vi "Sample - Add Speciment (SubVI).vi"(6 "Load?":bool, 7 "ID":string, 8 "error in":errorcluster, 9 "Data":string[](array[string]), 11 "JobID":string) -> (0 "error in 2":errorcluster, 3 "body":string)   [LabVIEW 2019]
uses:
  <vilib>/httpClient/POSTBuffer.vi
  <vilib>/httpClient/LabVIEWHTTPClient.lvlib
panel:
  in  "Type":enum16{"Circular", "Cubical"}(ring) caption="Enum 3"
  in  "Save":bool
  in  "Weight (g)":dbl format="%.2f"
  in  "Diameter/Length (mm)":dbl format="%.2f"
  in  "Height (mm)":dbl format="%.2f"
  in  "Depth (m)":dbl format="%.2f"
  in  "Specimen No":string
  in  "Sample No":string
  # "Specimen Details"
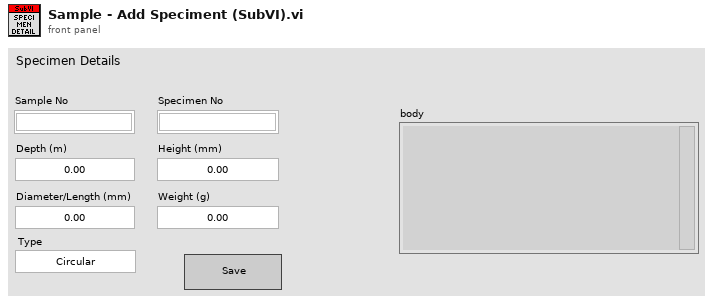
[diagram p1: front panel]
types:
  T1 = cluster{"action":string, "sampleno":string, "specimentno":string, "weight":string, "height":string, "depth":string, "diameter":string, "id":string, "jobid":string, "attribute":string}
  T2 = cluster{"action":string, "jobid":string, "sampleno":string, "specimentno":string, "weight":string, "height":string, "depth":string, "diameter":string, "attribute":string}
  T3 = typedef "LabVIEWHTTPClient.lvlib/ClientHandle.ctl" = refnum<k1>
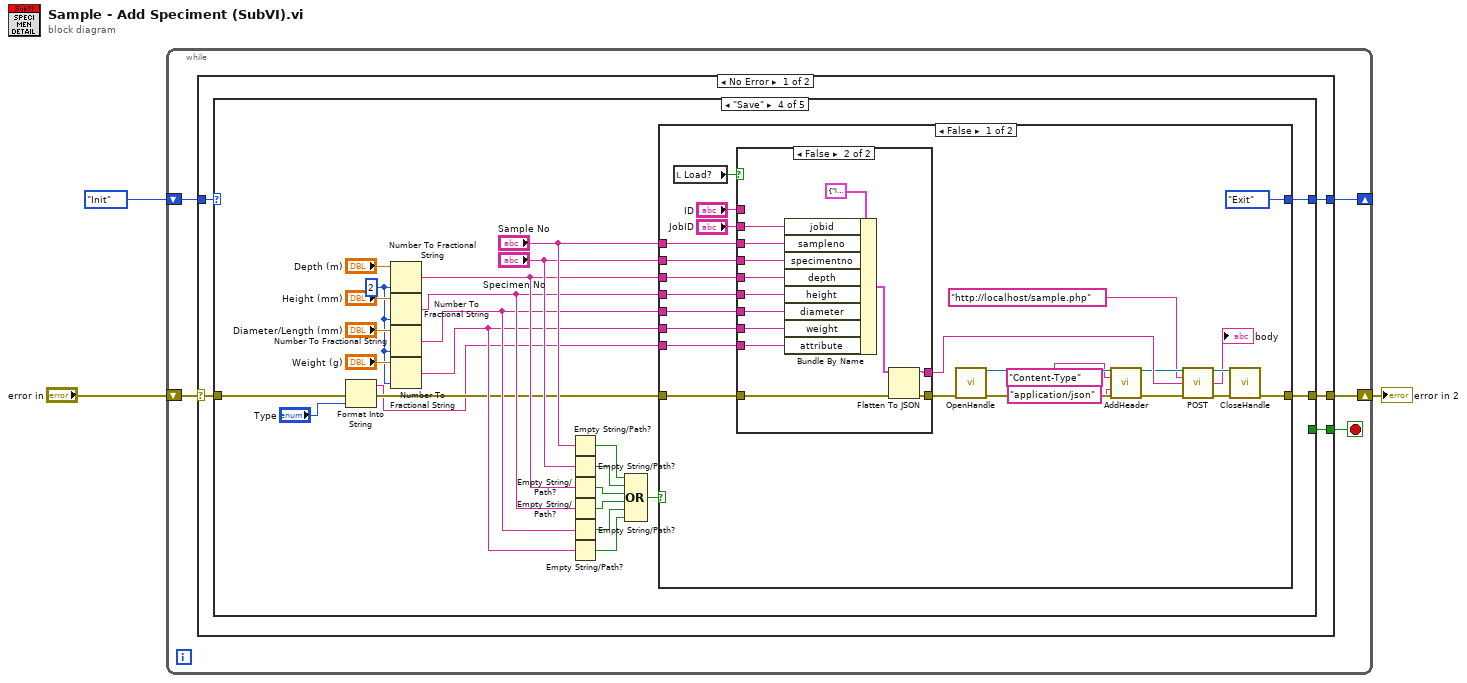
[diagram p0: block diagram]
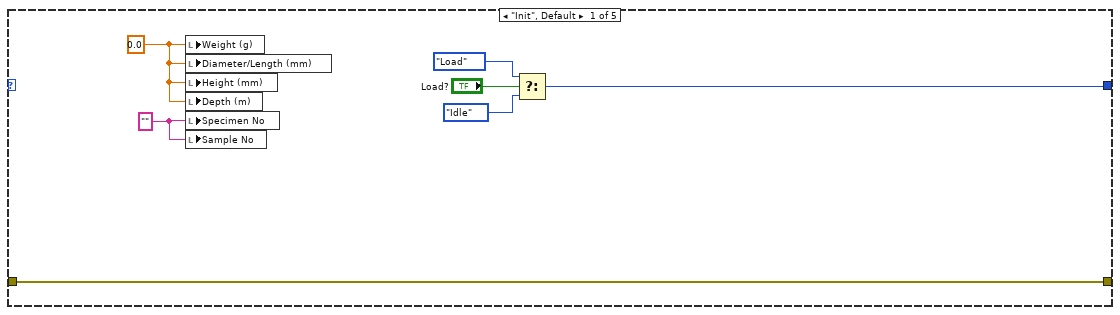
[diagram p2: hidden frame]
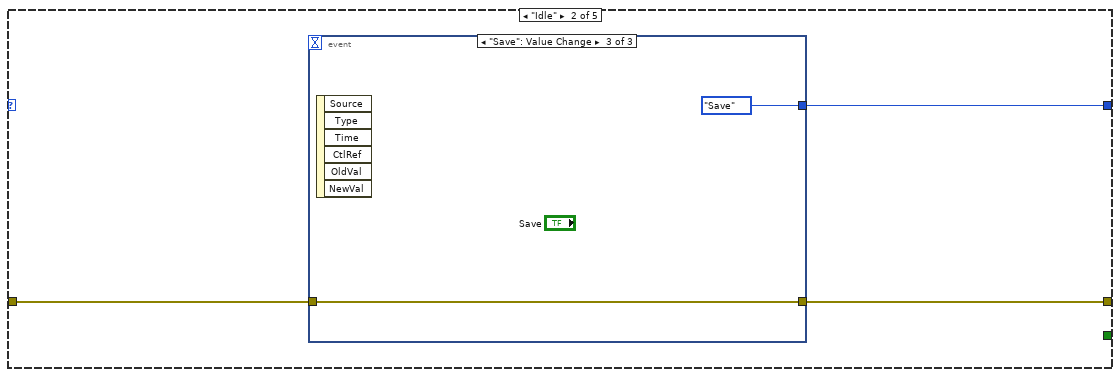
[diagram p3: hidden frame]
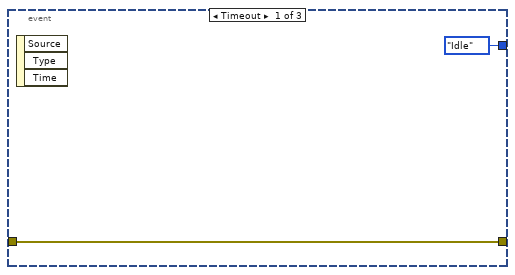
[diagram p4: hidden frame]
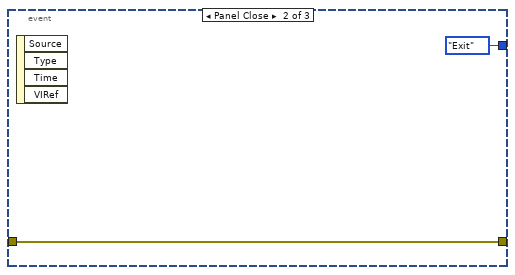
[diagram p5: hidden frame]
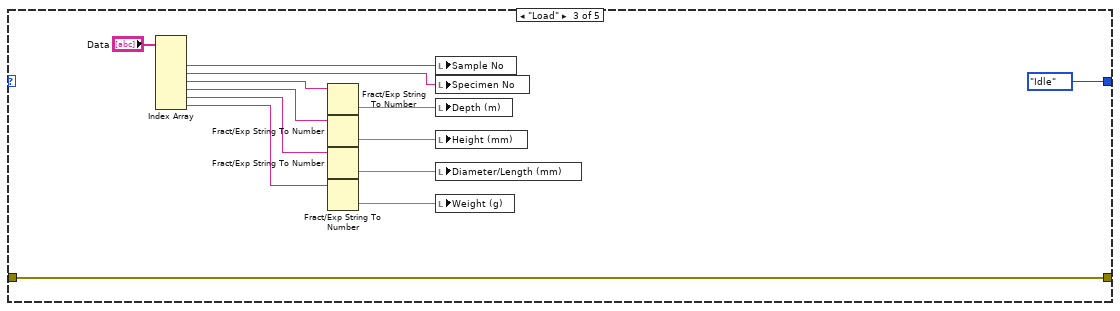
[diagram p6: hidden frame]
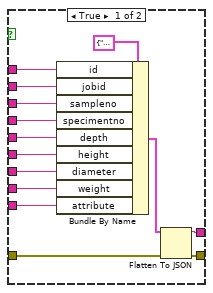
[diagram p7: hidden frame]
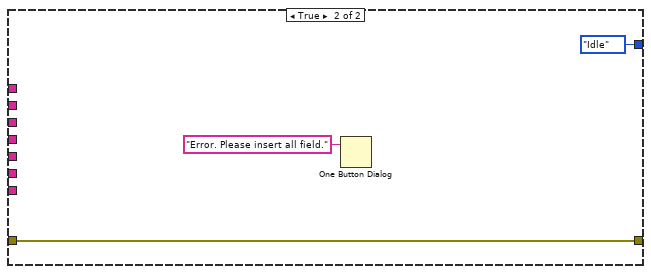
[diagram p8: hidden frame]
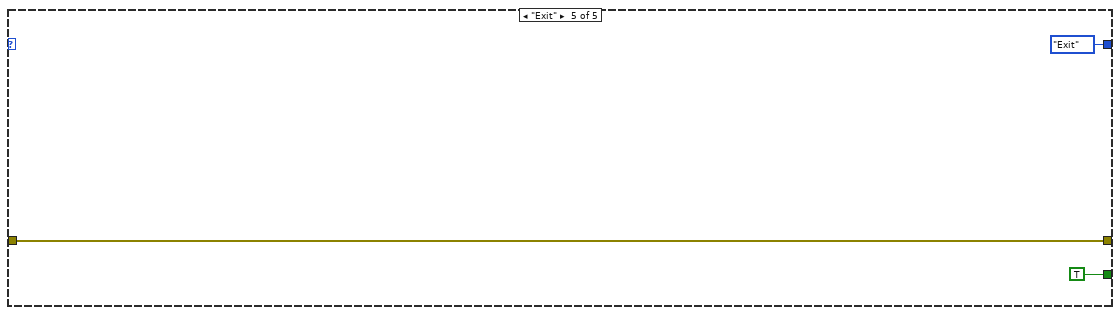
[diagram p9: hidden frame]
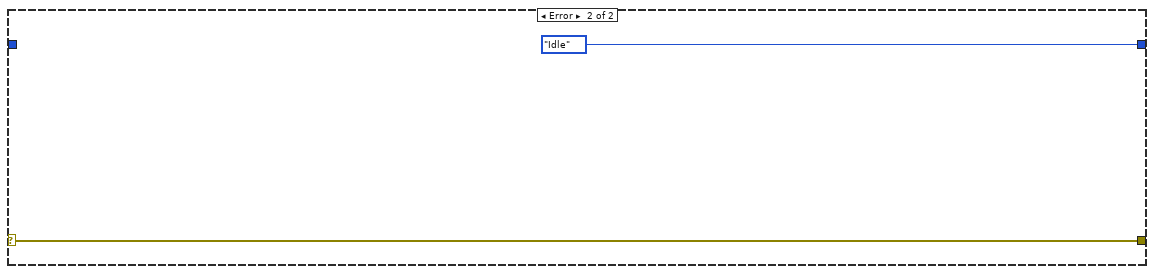
[diagram p10: hidden frame]
diagram:
  n1 = while {
    shift-right: [w6] -> w1
    shift-left: "error in" -> [w8]
    shift-right: [w5] -> _
    shift-left: enum16{"Init", "Idle", "Load", "Save", "Exit"}."Init" -> [w7]
    stop <- w4 stop-if-true
    n2 = case shown="No Error" w8 {
      selector: w8 -> [w11 w126]
      tunnel: w7 -> [w13 _]
      tunnel: [w12 w126] -> w6
      tunnel: [w10 enum16{"Init", "Idle", "Load", "Save", "Exit"}."Idle"] -> w5
      tunnel: [w9 _] -> w4
      frame No Error {
        n3 = case shown="\"Save\"" w13 {
          tunnel: [w20 w23 w42 w65 w124] -> w12
          tunnel: w11 -> [w20 w22 w42 w45 w124]
          tunnel: [w16 w21 enum16{"Init", "Idle", "Load", "Save", "Exit"}."Idle" ("f") w66 enum16{"Init", "Idle", "Load", "Save", "Exit"}."Exit" ("f")] -> w10
          tunnel: [_ _ _ _ TRUE] -> w9
          frame "Init", Default {
            w14 = 0.0 ("Weight (g)")
            w19 = "" ("Weight (g)")
            n4 = local write "Weight (g)"(w14) -> ()
            n5 = local write "Diameter/Length (mm)"(w14) -> ()
            n6 = local write "Height (mm)"(w14) -> ()
            n7 = local write "Depth (m)"(w14) -> ()
            n8 = local write "Specimen No"(w19) -> ()
            n9 = local write "Sample No"(w19) -> ()
            n10 = Select(t=enum16{"Init", "Idle", "Load", "Save", "Exit"}."Load", s="Load?", f=enum16{"Init", "Idle", "Load", "Save", "Exit"}."Idle") -> (s? t:f=w16:enum16{"Init", "Idle", "Load", "Save", "Exit"})
          }
          frame "Idle" {
            n11 = event shown="[2] \"Save\": Value Change" {
              selector: _ -> [_ _ _]
              dyn-events: _ -> [_ _ _]
              timeout: _ -> [_ _ _]
              tunnel: [w25 w26 w28] -> w23
              tunnel: w22 -> [w25 w26 w28]
              tunnel: [enum16{"Init", "Idle", "Load", "Save", "Exit"}."Idle" enum16{"Init", "Idle", "Load", "Save", "Exit"}."Exit" enum16{"Init", "Idle", "Load", "Save", "Exit"}."Save"] -> w21
              event Timeout {
                n12 = event-data() -> ()  [unwired: 1 in, 3 out]
              }
              event Panel Close {
                n13 = event-data() -> ()  [unwired: 1 in, 4 out]
              }
              event "Save": Value Change {
                n14 = event-data() -> ()  [unwired: 1 in, 6 out]
              }
            }
          }
          frame "Load" {
            n15 = Index Array(array="Data") -> (element #2=w39:string, element #3=w38:string, element #4=w37:string, element #5=w36:string, element #6=w35:string, element #7=w34:string)  [unwired: 7 in, 1 out]
            n16 = Fract/Exp String To Number(string=w37) -> (number=w33:dbl)  [unwired: 3 in, 1 out]
            n17 = Fract/Exp String To Number(string=w36) -> (number=w32:dbl)  [unwired: 3 in, 1 out]
            n18 = Fract/Exp String To Number(string=w35) -> (number=w31:dbl)  [unwired: 3 in, 1 out]
            n19 = Fract/Exp String To Number(string=w34) -> (number=w30:dbl)  [unwired: 3 in, 1 out]
            n20 = local write "Sample No"(w39) -> ()
            n21 = local write "Specimen No"(w38) -> ()
            n22 = local write "Depth (m)"(w33) -> ()
            n23 = local write "Height (mm)"(w32) -> ()
            n24 = local write "Diameter/Length (mm)"(w31) -> ()
            n25 = local write "Weight (g)"(w30) -> ()
          }
          frame "Save" {
            w47 = i16 2 ("precision (6)")
            n26 = Format Into String(error in=w45, "Type") -> (resulting string=w43:string, error out=w46:errorcluster)  [unwired: 2 in]
            n27 = Number To Fractional String(number="Depth (m)", precision (6)=w47) -> (F-format string=w58:string)  [unwired: 2 in]
            n28 = Number To Fractional String(number="Height (mm)", precision (6)=w47) -> (F-format string=w57:string)  [unwired: 2 in]
            n29 = Number To Fractional String(number="Diameter/Length (mm)", precision (6)=w47) -> (F-format string=w56:string)  [unwired: 2 in]
            n30 = Number To Fractional String(number="Weight (g)", precision (6)=w47) -> (F-format string=w55:string)  [unwired: 2 in]
            n31 = Empty String/Path?(string/path="Sample No") -> (empty?=w54:bool)
            n32 = Empty String/Path?(string/path="Specimen No") -> (empty?=w53:bool)
            n33 = Empty String/Path?(string/path=w58) -> (empty?=w52:bool)
            n34 = Empty String/Path?(string/path=w57) -> (empty?=w51:bool)
            n35 = Empty String/Path?(string/path=w56) -> (empty?=w50:bool)
            n36 = Empty String/Path?(string/path=w55) -> (empty?=w49:bool)
            n37 = Compound Arithmetic op=OR(w54, w53, w52, w51, w50, w49) -> (w48:bool)
            n38 = case shown="False" w48 {
              tunnel: [enum16{"Init", "Idle", "Load", "Save", "Exit"}."Exit" ("f") enum16{"Init", "Idle", "Load", "Save", "Exit"}."Idle" ("f")] -> w66
              tunnel: w46 -> [w79 w121]
              tunnel: [w78 w121] -> w65
              tunnel: "Sample No" -> [w73 _]
              tunnel: "Specimen No" -> [w72 _]
              tunnel: w58 -> [w71 _]
              tunnel: w57 -> [w70 _]
              tunnel: w56 -> [w69 _]
              tunnel: w55 -> [w68 _]
              tunnel: w43 -> [w67 _]
              frame False {
                n39 = local read "Load?"() -> (w76:bool)
                n40 = case shown="False" w76 {
                  tunnel: "ID" -> [w105 _]
                  tunnel: "JobID" -> [w104 w118]
                  tunnel: [w102 w116] -> w89
                  tunnel: w79 -> [w101 w115]
                  tunnel: [w100 w114] -> w90
                  tunnel: w73 -> [w99 w113]
                  tunnel: w72 -> [w98 w112]
                  tunnel: w71 -> [w97 w111]
                  tunnel: w70 -> [w96 w110]
                  tunnel: w69 -> [w95 w109]
                  tunnel: w68 -> [w94 w108]
                  tunnel: w67 -> [w92 w106]
                  frame True {
                    n41 = Bundle By Name(cluster=T1 {"action"="update", "sampleno"="", "specimentno"="", "weight"="", "height"="", "depth"="", "diameter"="", "id"="", "jobid"="", "attribute"=""}, "id"=w105, "jobid"=w104, "sampleno"=w99, "specimentno"=w98, "depth"=w97, "height"=w96, "diameter"=w95, "weight"=w94, "attribute"=w92) -> (w103:T1)
                    n42 = Flatten To JSON(anything=w103, error in (no error)=w101) -> (JSON string=w102:string, 11:w100:errorcluster)  [unwired: 1 in]
                  }
                  frame False {
                    n43 = Bundle By Name(cluster=T2 {"action"="insert", "jobid"="", "sampleno"="", "specimentno"="", "weight"="", "height"="", "depth"="", "diameter"="", "attribute"=""}, "jobid"=w118, "sampleno"=w113, "specimentno"=w112, "depth"=w111, "height"=w110, "diameter"=w109, "weight"=w108, "attribute"=w106) -> (w117:T2)
                    n44 = Flatten To JSON(anything=w117, error in (no error)=w115) -> (JSON string=w116:string, 11:w114:errorcluster)  [unwired: 1 in]
                  }
                }
                n45 = call <vilib>:"OpenHandle.vi"("error in (no error)"=w90) -> ("client handle out"=w86:T3, "error out"=w88:errorcluster)  [unwired: 13 in]
                n46 = call <vilib>:"AddHeader.vi"("client handle"=w86, "header"="Content-Type", "value"="application/json", "error in (no error)"=w88) -> ("client handle out"=w85:T3, "error out"=w87:errorcluster)  [unwired: 10 in]
                n47 = call-poly <vilib>:"POST.vi"("client handle"=w85, "url"="http://localhost/sample.php", "buffer"=w89, "error in (no error)"=w87) -> ("client handle out"=w83:T3, "body"=→"body":string, "error out"=w84:errorcluster)  [unwired: 8 in, 1 out]
                n48 = call <vilib>:"CloseHandle.vi"("client handle"=w83, "error in (no error)"=w84) -> ("error out"=w78:errorcluster)  [unwired: 13 in]
              }
              frame True {
                n49 = One Button Dialog(message="Error. Please insert all field.") -> ()  [unwired: 1 in, 1 out]
              }
            }
          }
          frame "Exit" {
          }
        }
      }
      frame Error {
      }
    }
  }
  "error in 2" <- w1
